vi "Pulse Generation (178x Smart Camera).vi"() -> ()   [LabVIEW 2023]
doc: "The Pulse Generation (178x Smart Camera) example perfoms pulse configuration on the user-selected pulse generator. The configuration can be updated at run-time."
uses:
  <vilib>/vision/driver/NI_Vision_Acquisition_Software.lvlib
  <resource>/objmgr/imaqdx.rc
panel:
  in  "Stop":bool
  in  "Pulse Selector":string(combo)="Pulse Generator 0"
  in  "Camera Name":refnum<k21> caption="IMAQdx Session"
  in  "SW Trigger":bool
  in  "Pulse Configuration":T1={"Mode"="Rearmed Pulse", "Polarity"="Active High", "Delay (us)"=1000.0, "Duration (us)"=1000.0, "Trigger Source"="Software", "Trigger Activation"="Rising Edge", "Delay Source"="Internal Clock", "Delay Edge Activation"="Rising Edge", "Delay Edge Counts"=3}
  # "Overview: Demonstrates how to use the pulse capabilities of the output lines on a ISC-178x smart camera.\nRequirements: Vision Acquisition Software, a ISC-178x smart camera.\nInstructions: \n1. Open a new LabVIEW Project by selecting Project»Create Project. Select Add this VI when prompted to add this VI to the project.\n2. Right click on the top-level project item in the tree and select New»Targets and Devices\n3. Select the ISC-178x smart camera you want to run this example with, and click OK.\n4. Drag this VI from My Computer to the smart camera target.\n5. Double click on the example under the smart camera, select the Camera Name, and run the VI."
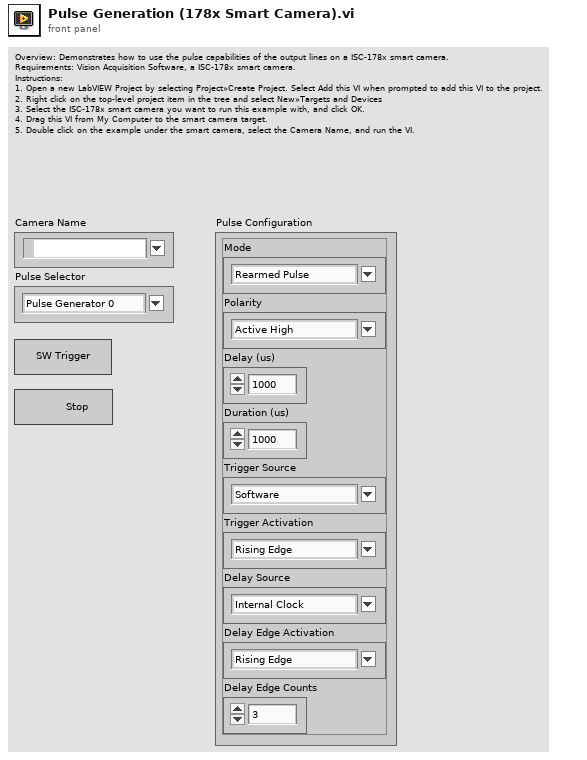
[diagram p1: front panel]
types:
  T1 = cluster{"Mode":string, "Polarity":string, "Delay (us)":dbl, "Duration (us)":dbl, "Trigger Source":string, "Trigger Activation":string, "Delay Source":string, "Delay Edge Activation":string, "Delay Edge Counts":u32}
  T2 = typedef "IMAQdx.ctl" = refnum<k21>
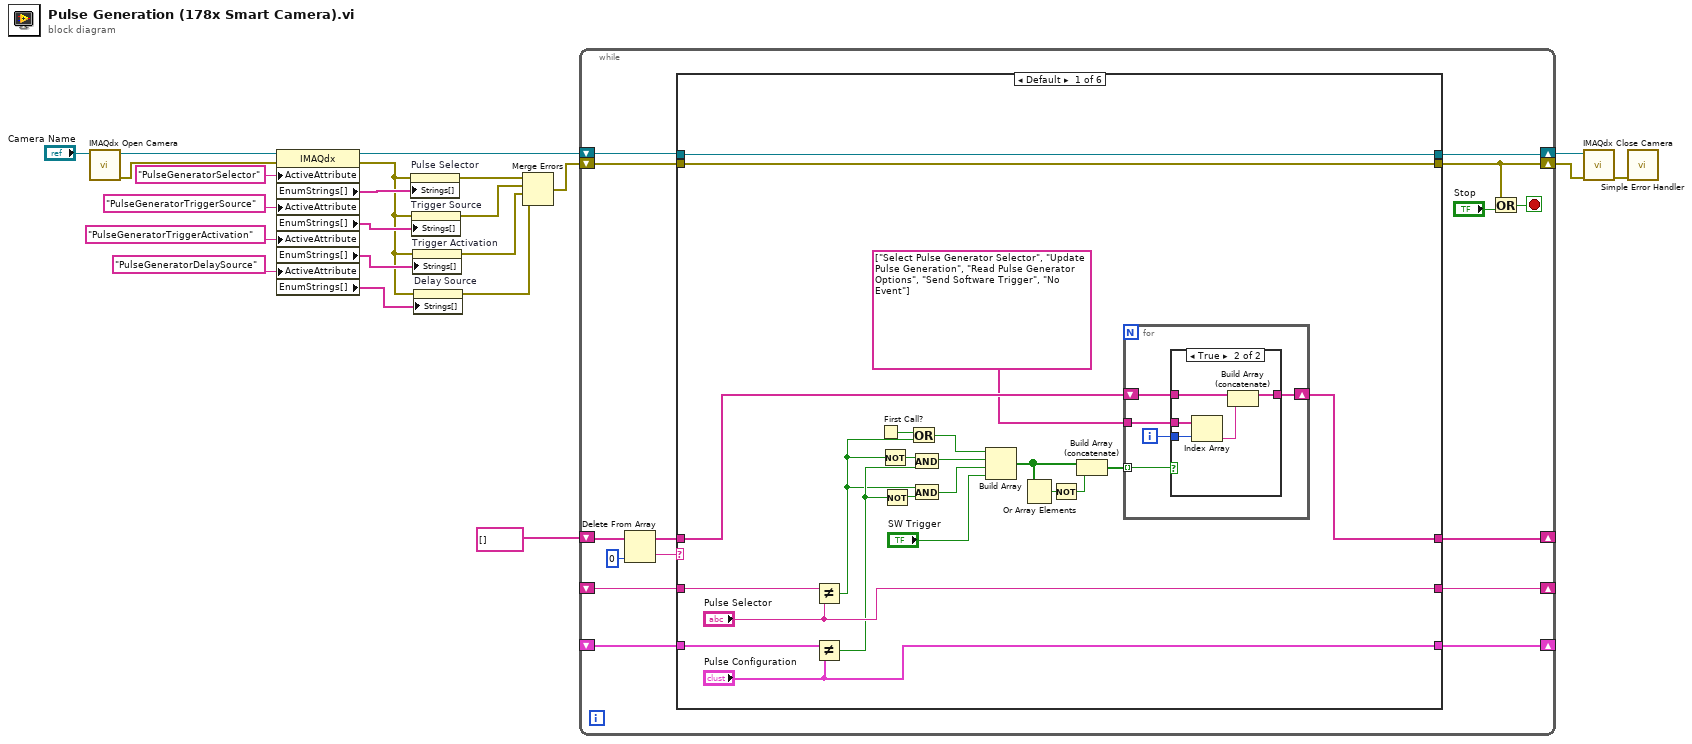
[diagram p0: block diagram]
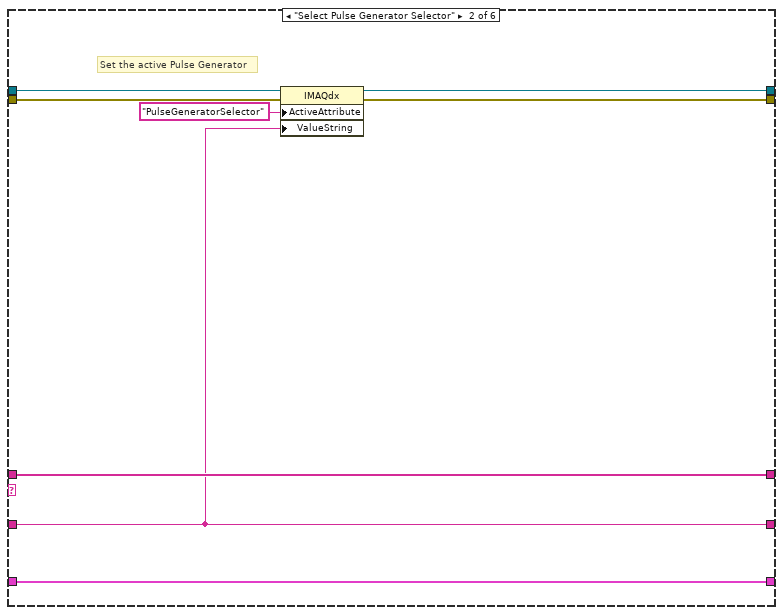
[diagram p3: hidden frame]
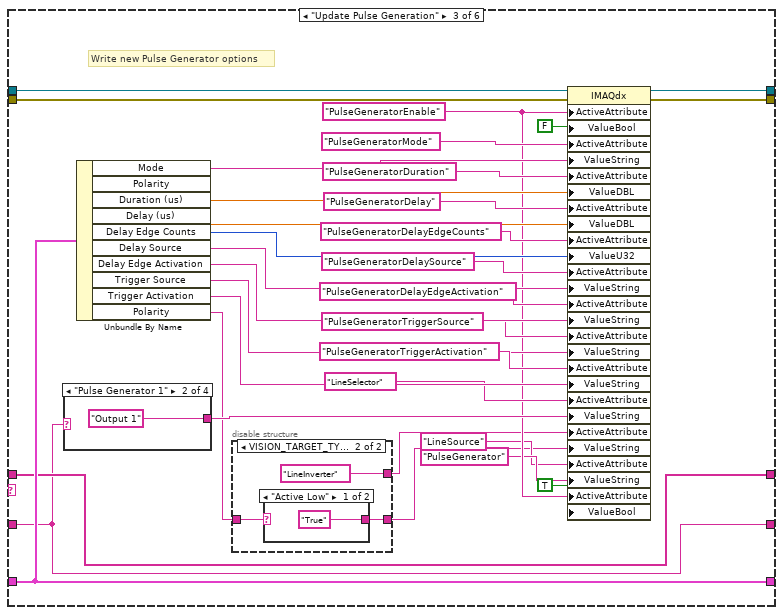
[diagram p4: hidden frame]
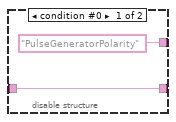
[diagram p5: hidden frame]
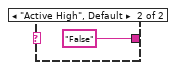
[diagram p6: hidden frame]
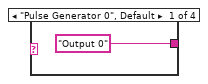
[diagram p7: hidden frame]
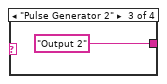
[diagram p8: hidden frame]
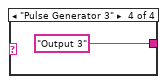
[diagram p9: hidden frame]
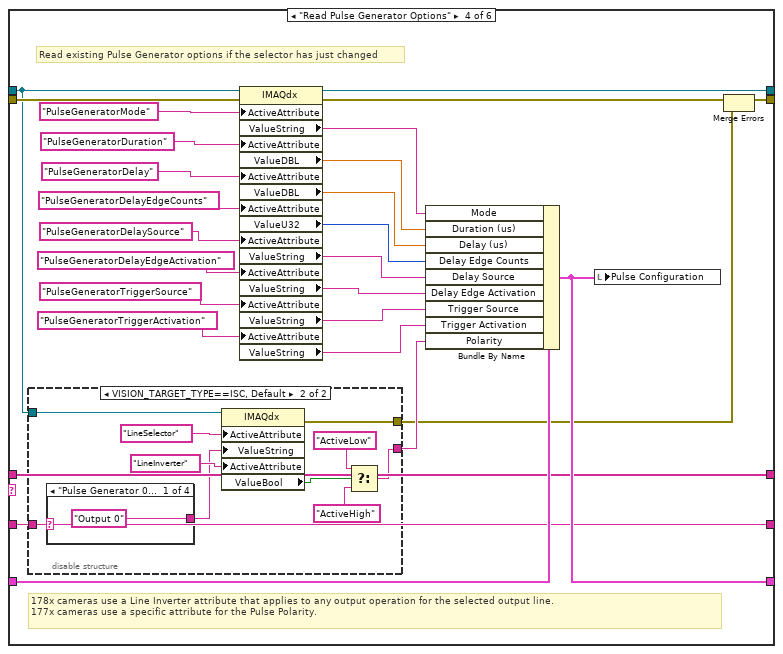
[diagram p10: hidden frame]
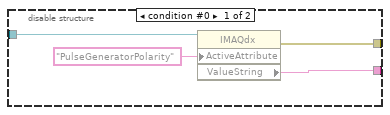
[diagram p11: hidden frame]
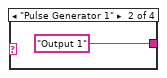
[diagram p12: hidden frame]
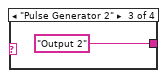
[diagram p13: hidden frame]
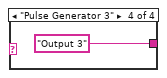
[diagram p14: hidden frame]
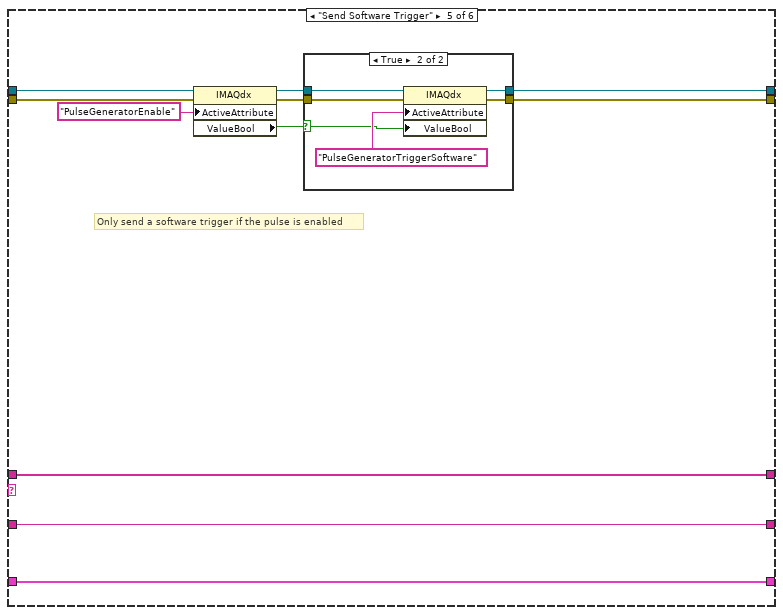
[diagram p15: hidden frame]
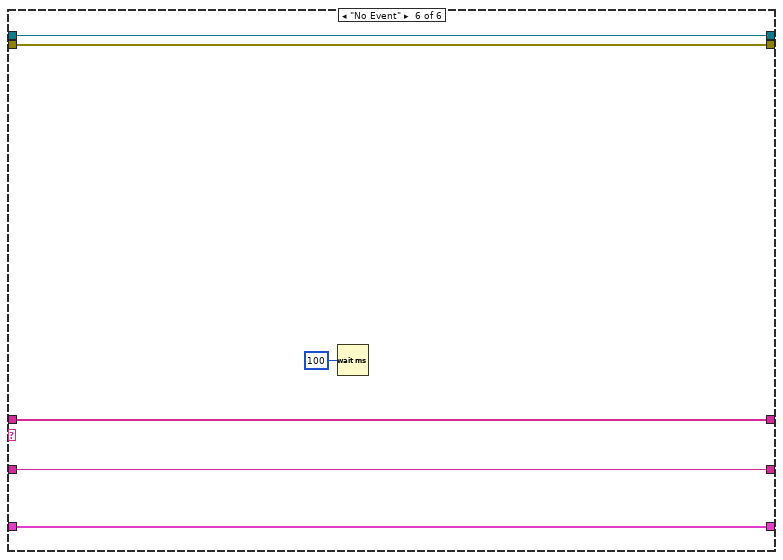
[diagram p17: hidden frame]
diagram:
  n1 = call <vilib>:"IMAQdx Open Camera.vi"("Session In"="Camera Name") -> ("error out"=w16:errorcluster, "Session Out"=w17:T2)  [unwired: 2 in, 7 out]
  n2 = property class="IMAQdx"(reference=w17, error in=w16, "ActiveAttribute"="PulseGeneratorSelector", "ActiveAttribute"="PulseGeneratorTriggerSource", "ActiveAttribute"="PulseGeneratorTriggerActivation", "ActiveAttribute"="PulseGeneratorDelaySource") -> (reference out=w15:T2, error out=w2:errorcluster, "EnumStrings[]"=w13:string[], "EnumStrings[]"=w11:string[], "EnumStrings[]"=w9:string[], "EnumStrings[]"=w3:string[])
  n3 = property on="Pulse Selector" class="CmbBox"(error in=w2, "Strings[]"=w13) -> (error out=w8:errorcluster)  [unwired: 1 in, 1 out]
  n4 = property on="Trigger Source" class="CmbBox"(error in=w2, "Strings[]"=w11) -> (error out=w7:errorcluster)  [unwired: 1 in, 1 out]
  n5 = property on="Trigger Activation" class="CmbBox"(error in=w2, "Strings[]"=w9) -> (error out=w6:errorcluster)  [unwired: 1 in, 1 out]
  n6 = property on="Delay Source" class="CmbBox"(error in=w2, "Strings[]"=w3) -> (error out=w5:errorcluster)  [unwired: 1 in, 1 out]
  n7 = Merge Errors(w8, w7, w6, w5) -> (w4:errorcluster)
  n8 = while {
    shift-right: [w25] -> _
    shift-left: _ -> [w26]
    shift-right: [w35] -> _
    shift-left: _ -> [w24]
    shift-right: [w32] -> w21
    shift-left: w15 -> [w37]
    shift-right: [w31] -> w20
    shift-left: w4 -> [w36]
    shift-right: [w27] -> _
    shift-left: string[] [] -> [w29]
    stop <- w33 stop-if-true
    n9 = Delete From Array(array=w29, index=0) -> (deleted portion=w23:string, array with subset deleted=w28:string[])  [unwired: 1 in]
    n10 = case shown="Default" w23 {
      tunnel: w37 -> [w59 w77 w111 w128 w174 w191]
      tunnel: w36 -> [w58 w76 w110 w149 w173 w190]
      tunnel: [w59 w75 w109 w148 w172 w191] -> w32
      tunnel: [w58 w74 w90 w124 w171 w190] -> w31
      tunnel: ["Pulse Configuration" w71 w89 w147 w168 w187] -> w35
      tunnel: w28 -> [w53 w73 w88 w129 w170 w189]
      tunnel: [w51 w73 w88 w129 w170 w189] -> w27
      tunnel: w26 -> [w49 w72 w86 w123 w169 w188]
      tunnel: ["Pulse Selector" w72 w86 w123 w169 w188] -> w25
      tunnel: w24 -> [w45 w71 w89 w130 w168 w187]
      frame Default {
        n11 = Not Equal?(x=w49, y="Pulse Selector") -> (x != y?=w38:bool)
        n12 = Not Equal?(x=w45, y="Pulse Configuration") -> (x != y?=w40:bool)
        n13 = First Call?() -> (First Call?: T/F=w47:bool)
        n14 = Not(x=w38) -> (.not. x?=w44:bool)
        n15 = Not(x=w40) -> (.not. x?=w39:bool)
        n16 = Or(x=w47, y=w38) -> (x .or. y?=w46:bool)
        n17 = And(x=w44, y=w40) -> (x .and. y?=w42:bool)
        n18 = And(x=w38, y=w39) -> (x .and. y?=w41:bool)
        n19 = Build Array(w46, w42, w41, "SW Trigger") -> (w54:bool[])
        n20 = Or Array Elements(Boolean array=w54) -> (logical OR=w56:bool)
        n21 = Not(x=w56) -> (.not. x?=w57:bool)
        n22 = Build Array (concatenate)(w54, w57) -> (w55:bool[])
        n23 = for {
          tunnel: w55 -> [w64] mode=indexing
          shift-right: [w62] -> w51
          shift-left: w53 -> [w63]
          tunnel: string[] ["Select Pulse Generator Selector", "Update Pulse Generation", "Read Pulse Generator Options", "Send Software Trigger", "No Event"] -> [w61]
          i -> [w60]
          n24 = case shown="True" w64 {
            tunnel: w63 -> [w65 w70]
            tunnel: w60 -> [_ w69]
            tunnel: [w65 w67] -> w62
            tunnel: w61 -> [_ w66]
            frame False {
            }
            frame True {
              n25 = Index Array(array=w66, index=w69) -> (element=w68:string)
              n26 = Build Array (concatenate)(w70, w68) -> (w67:string[])
            }
          }
        }
      }
      frame "Select Pulse Generator Selector" {
        # "Set the active Pulse Generator"
        n27 = property class="IMAQdx"(reference=w77, error in=w76, "ActiveAttribute"="PulseGeneratorSelector", "ValueString"=w72) -> (reference out=w75:T2, error out=w74:errorcluster)
      }
      frame "Update Pulse Generation" {
        w84 = "PulseGeneratorEnable" ("ActiveAttribute")
        # "Write new Pulse Generator options"
        n28 = case shown="\"Pulse Generator 1\"" w86 {
          tunnel: ["Output 0" "Output 1" "Output 2" "Output 3"] -> w91
          frame "Pulse Generator 0", Default {
          }
          frame "Pulse Generator 1" {
          }
          frame "Pulse Generator 2" {
          }
          frame "Pulse Generator 3" {
          }
        }
        n29 = Unbundle By Name(w89) -> ("Mode"=w106:string, "Duration (us)"=w104:dbl, "Delay (us)"=w102:dbl, "Delay Edge Counts"=w87:u32, "Delay Source"=w99:string, "Delay Edge Activation"=w97:string, "Trigger Source"=w94:string, "Trigger Activation"=w93:string, "Polarity"=w80:string)  [unwired: 1 out]
        n30 = disable-structure shown="VISION_TARGET_TYPE==ISC, Default" {
          disable-tunnel: ["PulseGeneratorPolarity" ("ActiveAttribute") "LineInverter" ("ActiveAttribute")] -> w81
          disable-tunnel: w80 -> [w112 w115]
          disable-tunnel: [w112 w114] -> w79
          frame condition #0 {
          }
          frame condition #1 (active) {
            n31 = case shown="\"Active Low\"" w115 {
              tunnel: ["True" "False"] -> w114
              frame "Active Low" {
              }
              frame "Active High", Default {
              }
            }
          }
        }
        n32 = property class="IMAQdx"(reference=w111, error in=w110, "ActiveAttribute"=w84, "ValueBool"=FALSE, "ActiveAttribute"="PulseGeneratorMode", "ValueString"=w106, "ActiveAttribute"="PulseGeneratorDuration", "ValueDBL"=w104, "ActiveAttribute"="PulseGeneratorDelay", "ValueDBL"=w102, "ActiveAttribute"="PulseGeneratorDelayEdgeCounts", "ValueU32"=w87, "ActiveAttribute"="PulseGeneratorDelaySource", "ValueString"=w99, "ActiveAttribute"="PulseGeneratorDelayEdgeActivation", "ValueString"=w97, "ActiveAttribute"="PulseGeneratorTriggerSource", "ValueString"=w94, "ActiveAttribute"="PulseGeneratorTriggerActivation", "ValueString"=w93, "ActiveAttribute"="LineSelector", "ValueString"=w91, "ActiveAttribute"=w81, "ValueString"=w79, "ActiveAttribute"="LineSource", "ValueString"="PulseGenerator" ("ActiveAttribute"), "ActiveAttribute"=w84, "ValueBool"=TRUE) -> (reference out=w109:T2, error out=w90:errorcluster)
      }
      frame "Read Pulse Generator Options" {
        # "178x cameras use a Line Inverter attribute that applies to any output operation for the selected output line.\n177x cameras use a specific attribute for the Pulse Polarity."
        # "Read existing Pulse Generator options if the selector has just changed"
        n33 = disable-structure shown="VISION_TARGET_TYPE==ISC, Default" {
          disable-tunnel: w128 -> [w153 w163]
          disable-tunnel: [w151 w154] -> w127
          disable-tunnel: [w150 w158] -> w125
          disable-tunnel: w123 -> [_ w160]
          frame condition #0 {
            n34 = property class="IMAQdx"(reference=w153, "ActiveAttribute"="PulseGeneratorPolarity") -> (error out=w150:errorcluster, "ValueString"=w151:string)  [unwired: 1 in, 1 out]
          }
          frame condition #1 (active) {
            n35 = case shown="\"Pulse Generator 0\", Default" w160 {
              tunnel: ["Output 0" "Output 1" "Output 2" "Output 3"] -> w159
              frame "Pulse Generator 0", Default {
              }
              frame "Pulse Generator 1" {
              }
              frame "Pulse Generator 2" {
              }
              frame "Pulse Generator 3" {
              }
            }
            n36 = property class="IMAQdx"(reference=w163, "ActiveAttribute"="LineSelector", "ValueString"=w159, "ActiveAttribute"="LineInverter") -> (error out=w158:errorcluster, "ValueBool"=w157:bool)  [unwired: 1 in, 1 out]
            n37 = Select(t="ActiveLow" ("ActiveAttribute"), s=w157, f="ActiveHigh" ("ActiveAttribute")) -> (s? t:f=w154:string)
          }
        }
        n38 = property class="IMAQdx"(reference=w128, error in=w149, "ActiveAttribute"="PulseGeneratorMode", "ActiveAttribute"="PulseGeneratorDuration", "ActiveAttribute"="PulseGeneratorDelay", "ActiveAttribute"="PulseGeneratorDelayEdgeCounts", "ActiveAttribute"="PulseGeneratorDelaySource", "ActiveAttribute"="PulseGeneratorDelayEdgeActivation", "ActiveAttribute"="PulseGeneratorTriggerSource", "ActiveAttribute"="PulseGeneratorTriggerActivation") -> (reference out=w148:T2, error out=w126:errorcluster, "ValueString"=w139:string, "ValueDBL"=w138:dbl, "ValueDBL"=w137:dbl, "ValueU32"=w136:u32, "ValueString"=w135:string, "ValueString"=w134:string, "ValueString"=w133:string, "ValueString"=w132:string)
        n39 = Bundle By Name(cluster=w130, "Mode"=w139, "Duration (us)"=w138, "Delay (us)"=w137, "Delay Edge Counts"=w136, "Delay Source"=w135, "Delay Edge Activation"=w134, "Trigger Source"=w133, "Trigger Activation"=w132, "Polarity"=w127) -> (w147:T1)
        n40 = local write "Pulse Configuration"(w147) -> ()
        n41 = Merge Errors(w126, w125) -> (w124:errorcluster)
      }
      frame "Send Software Trigger" {
        # "Only send a software trigger if the pulse is enabled"
        n42 = property class="IMAQdx"(reference=w174, error in=w173, "ActiveAttribute"="PulseGeneratorEnable") -> (reference out=w175:T2, error out=w176:errorcluster, "ValueBool"=w178:bool)
        n43 = case shown="True" w178 {
          selector: w178 -> [_ w181]
          tunnel: [w180 w186] -> w172
          tunnel: [w179 w185] -> w171
          tunnel: w175 -> [w180 w183]
          tunnel: w176 -> [w179 w182]
          frame False {
          }
          frame True {
            n44 = property class="IMAQdx"(reference=w183, error in=w182, "ActiveAttribute"="PulseGeneratorTriggerSoftware", "ValueBool"=w181) -> (reference out=w186:T2, error out=w185:errorcluster)
          }
        }
      }
      frame "No Event" {
        n45 = Wait (ms)(milliseconds to wait=u32 100 ("millisecond multiple")) -> ()  [unwired: 1 out]
      }
    }
    n46 = Or(x=w31, y="Stop") -> (x .or. y?=w33:bool)
  }
  n47 = call <vilib>:"IMAQdx Close Camera.vi"("error in"=w20, "Session In"=w21) -> ("error out"=w19:errorcluster)  [unwired: 9 out]
  n48 = call <vilib>:"Simple Error Handler.vi"("error in (no error)"=w19) -> ()  [unwired: 1 in, 8 out]
